vi "average waveform.vi"(7 "DAQ cluster in":T1 {"temp"."utility"."therm volt" format="%_6g"; "temp"."utility"."heat volt in" format="%_6g"; "temp"."utility"."heat volt out" format="%_6g"; "temp"."utility"."power out" format="%_6g"; "temp"."utility"."H Vmax" format="%_6g"; "temp"."T exec"."man power" format="%_6g"; "temp"."T exec"."exec setpoint" format="%_6g"; "temp"."T params"."Settle Time" step=1.0; "temp"."T params"."Settle Bandwidth" step=0.01; "temp"."T params"."Derivative Tme" step=0.01; "temp"."T params"."Integral Time" step=1.0; "temp"."T params"."Control Bandwidth" step=0.1; "temp"."T params"."Setpoint" step=0.1; "temp"."T status"."Setpoint" format="%_6g"; "temp"."T status"."Power" format="%_6g"; "temp"."T status"."Temp" format="%_6g"}) -> (8 "DAQ cluster out":T1 {"temp"."utility"."therm volt" format="%_6g"; "temp"."utility"."heat volt in" format="%_6g"; "temp"."utility"."heat volt out" format="%_6g"; "temp"."utility"."power out" format="%_6g"; "temp"."utility"."H Vmax" format="%_6g"; "temp"."T exec"."man power" format="%_6g"; "temp"."T exec"."exec setpoint" format="%_6g"; "temp"."T params"."Settle Time" step=1.0; "temp"."T params"."Settle Bandwidth" step=0.01; "temp"."T params"."Derivative Tme" step=0.01; "temp"."T params"."Integral Time" step=1.0; "temp"."T params"."Control Bandwidth" step=0.1; "temp"."T params"."Setpoint" step=0.1; "temp"."T status"."Setpoint" format="%_6g"; "temp"."T status"."Power" format="%_6g"; "temp"."T status"."Temp" format="%_6g"})   [LabVIEW 2019]
doc: "This is a Bug C(T) subVI.\n\nThis subVI is one of the states of the DAQ state machine in the bug experiment.\n\nThis state performs a running average of the raw waveforms. It sets the \"avg complete\" flag when it reaches the num of avg repetitions.\n\nIt goes to global comm as its next state.\n \nPaul K Dixon\nP3600\nCSUSB Physics"
uses:
  typedefs/DAQ state cluster.ctl
  typedefs/DAQ state enum.ctl
  typedefs/temp cont cluster.ctl
  typedefs/temp exec cluster.ctl
  typedefs/temp mode enum.ctl
  typedefs/temp indicator.ctl
  typedefs/temp control status.ctl
  typedefs/PID control parameters.ctl
  typedefs/temp cont utility.ctl
  typedefs/measurement.ctl
  typedefs/wvfm acq params.ctl
panel:
  out "avg complete":bool=TRUE
  out "meas index":i32=337
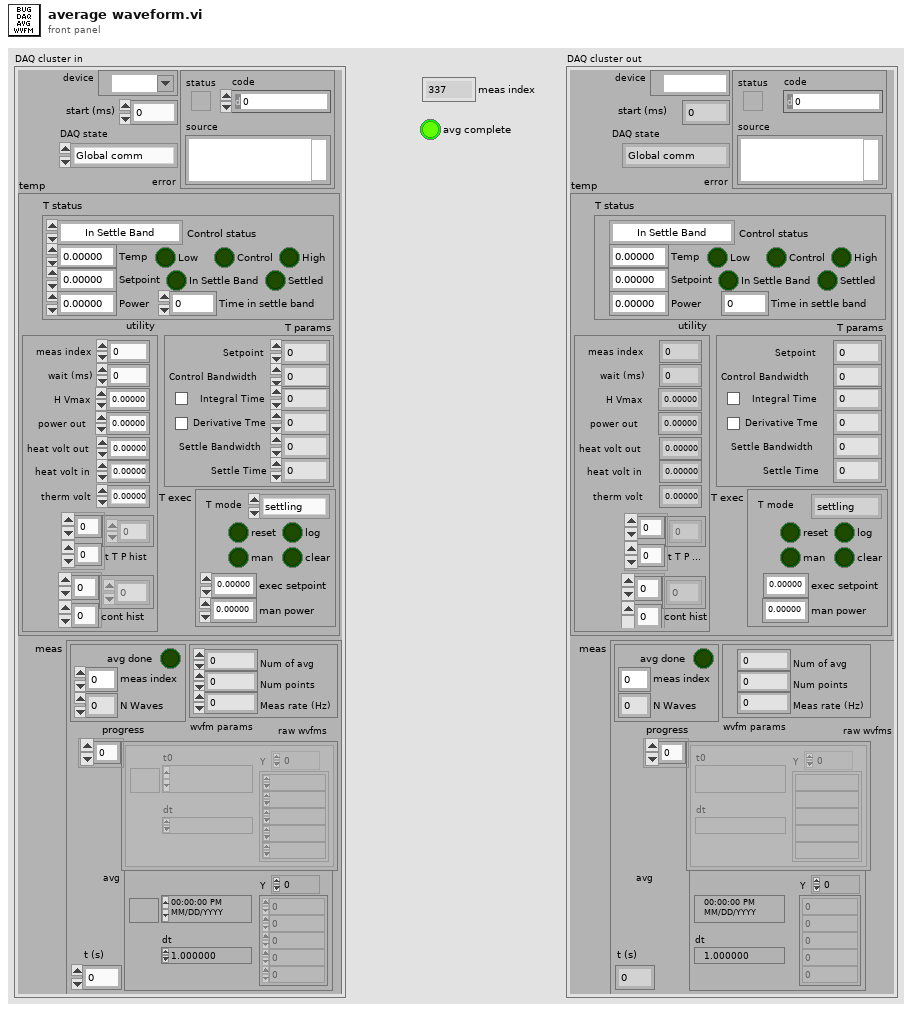
[diagram p1: front panel]
types:
  T1 = typedef "DAQ state cluster.ctl" = cluster{"DAQ state":T2, "temp":T3, "meas":T10, "device":tag, "error":errorcluster, "start (ms)":i32}
  T2 = typedef "DAQ state enum.ctl" = enum16{"Global comm", "Meas T & P", "PID power calc", "Man Power set", "Output Power", "Wait", "Meas wvfm", "Avg wvfm", "Exit"}
  T3 = typedef "temp cont cluster.ctl" = cluster{"T exec":T4, "T status":T6, "T params":T8, "utility":T9}
  T4 = typedef "temp exec cluster.ctl" = cluster{"T mode":T5, "exec setpoint":dbl, "reset":bool, "man power":dbl, "man":bool, "log":bool, "clear":bool}
  T5 = typedef "temp mode enum.ctl" = enum16{"settling", "measuring", "holding", "Exit"}
  T6 = typedef "temp indicator.ctl" = cluster{"Control status":T7, "Temp":dbl, "Power":dbl, "Time in settle band":dbl, "Settled":bool, "Low":bool, "High":bool, "Setpoint":dbl, "Control":bool, "In Settle Band":bool}
  T7 = typedef "temp control status.ctl" = enum16{"In Settle Band", "In Control Band", "Below Control Band", "Above Control Band"}
  T8 = typedef "PID control parameters.ctl" = cluster{"Setpoint":dbl, "Control Bandwidth":dbl, "Integral Time":dbl, "Int\nON":bool, "Derivative Tme":dbl, "Der\nON":bool, "Settle Bandwidth":dbl, "Settle Time":dbl}
  T9 = typedef "temp cont utility.ctl" = cluster{"meas index":i32, "wait (ms)":i32, "H Vmax":dbl, "power out":dbl, "heat volt out":dbl, "heat volt in":dbl, "therm volt":dbl, "t T P hist":dbl[][], "cont hist":dbl[][]}
  T10 = typedef "measurement.ctl" = cluster{"wvfm params":T11, "avg":waveform(dbl), "raw wvfms":waveform(dbl)[], "progress":cluster{"avg done":bool, "meas index":i32, "N waves":i32}, "t (s)":dbl}
  T11 = typedef "wvfm acq params.ctl" = cluster{"Num of avg":i32, "Num points":i32, "Meas rate (Hz)":dbl}
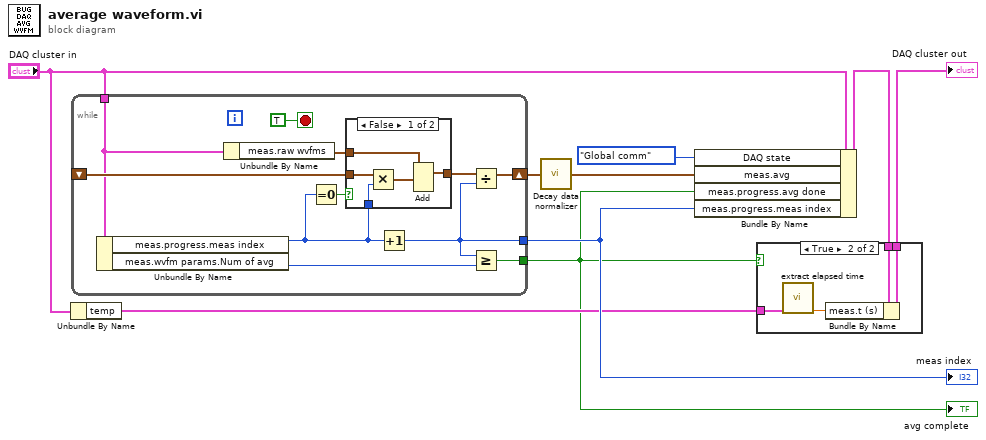
[diagram p0: block diagram]
diagram:
  n1 = Unbundle By Name("DAQ cluster in") -> ("temp"=w4:T3)
  n2 = while {
    shift-right: [w19] -> w7
    shift-left: _ -> [w18]
    tunnel: [w17] -> w3
    tunnel: [w12] -> w6
    tunnel: "DAQ cluster in" -> [w11]
    stop <- TRUE stop-if-true
    n3 = Unbundle By Name(w11) -> ("meas.progress.meas index"=w14:i32, "meas.wvfm params.Num of avg"=w13:i32)
    n4 = Unbundle By Name(w11) -> ("meas.raw wvfms"=w10:waveform(dbl)[])
    n5 = Equal To 0?(x=w14) -> (x = 0?=w15:bool)
    n6 = case shown="False" w15 {
      tunnel: w18 -> [w25 _]
      tunnel: w10 -> [w23 w26]
      tunnel: [w22 w26] -> w16
      tunnel: w14 -> [w21 _]
      frame False {
        n7 = Multiply(x=w25, y=w21) -> (x*y=w24:waveform(dbl)[])
        n8 = Add(1:w24, 2:w23) -> (0:w22:waveform(dbl)[])  [unwired: 1 in, 1 out]
      }
      frame True {
      }
    }
    n9 = Increment(x=w14) -> (x+1=w12:i32)
    n10 = Divide(x=w16, y=w12) -> (x/y=w19:waveform(dbl)[])
    n11 = Greater Or Equal?(x=w12, y=w13) -> (x >= y?=w17:bool)
  }
  "avg complete" <- w3
  "meas index" <- w6
  n12 = call "Decay data normalizer.vi"("avg wvfms"=w7) -> ("norm avg wave"=w8:waveform(dbl))  [unwired: 14 in]
  n13 = Bundle By Name(cluster="DAQ cluster in", "DAQ state"=DAQ_state_enum."Global comm", "meas.avg"=w8, "meas.progress.avg done"=w3, "meas.progress.meas index"=w6) -> (w2:T1)
  n14 = case shown="True" w3 {
    tunnel: w4 -> [_ w31]
    tunnel: w2 -> [w27 w29]
    tunnel: [w27 w28] -> w1
    frame False {
    }
    frame True {
      n15 = call "extract elapsed time.vi"("temp"=w31) -> ("latest time (s)"=w30:dbl)  [unwired: 14 in]
      n16 = Bundle By Name(cluster=w29, "meas.t (s)"=w30) -> (w28:T1)
    }
  }
  "DAQ cluster out" <- w1
